vi "distance to speed scaler.vi"(3 "Min Speed":dbl=1.0, 4 "Max Speed":dbl=5.0, 5 "Distance (mm)":i32=9) -> (1 "Speed (0..10)":dbl=5.0)   [LabVIEW 2017]
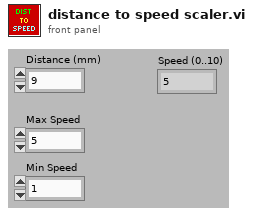
[diagram p1: front panel]
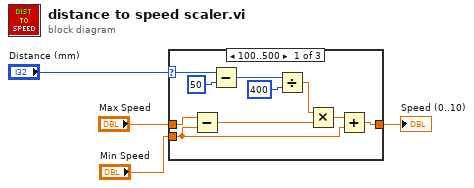
[diagram p0: block diagram]
diagram:
  n1 = case shown="100..500" "Distance (mm)" {
    selector: "Distance (mm)" -> [w11 _ _]
    tunnel: [w5 w15 w16] -> w4
    tunnel: "Max Speed" -> [w12 _ w16]
    tunnel: "Min Speed" -> [w13 w15 _]
    frame 100..500 {
      n2 = Subtract(x=w12, y=w13) -> (x-y=w7:dbl)
      n3 = Subtract(x=w11, y=50) -> (x-y=w9:i32)
      n4 = Divide(x=w9, y=400) -> (x/y=w8:dbl)
      n5 = Multiply(x=w8, y=w7) -> (x*y=w6:dbl)
      n6 = Add(x=w6, y=w13) -> (x+y=w5:dbl)
    }
    frame ..99 {
    }
    frame Default {
    }
  }
  "Speed (0..10)" <- w4
